vi "Results_filename_checker.vi"(4 "Filelength":i32=25, 5 "Warn if Already Exists":bool, 6 "Comment":string, 7 "Show Error handler":bool=TRUE, 8 "Results file":path) -> (0 "exists?":bool, 1 "Error String":string, 2 "cancelled":bool, 3 "Results file output":path)   [LabVIEW 2010]
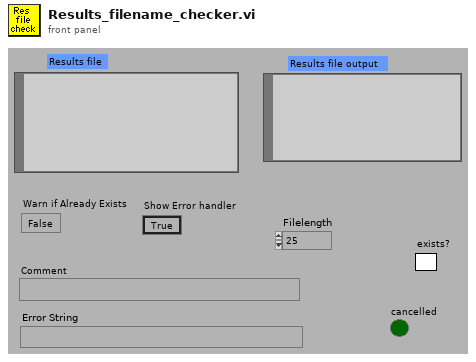
[diagram p1: front panel]
types:
  T1 = enum32{"existing file", "new file", "new or existing file", "existing dir", "new dir", "new or existing dir", "existing file (use LLBs)", "new file (use LLBs)", "new or existing file (use LLBs)", "new or existing file or directory (use LLBs)"}
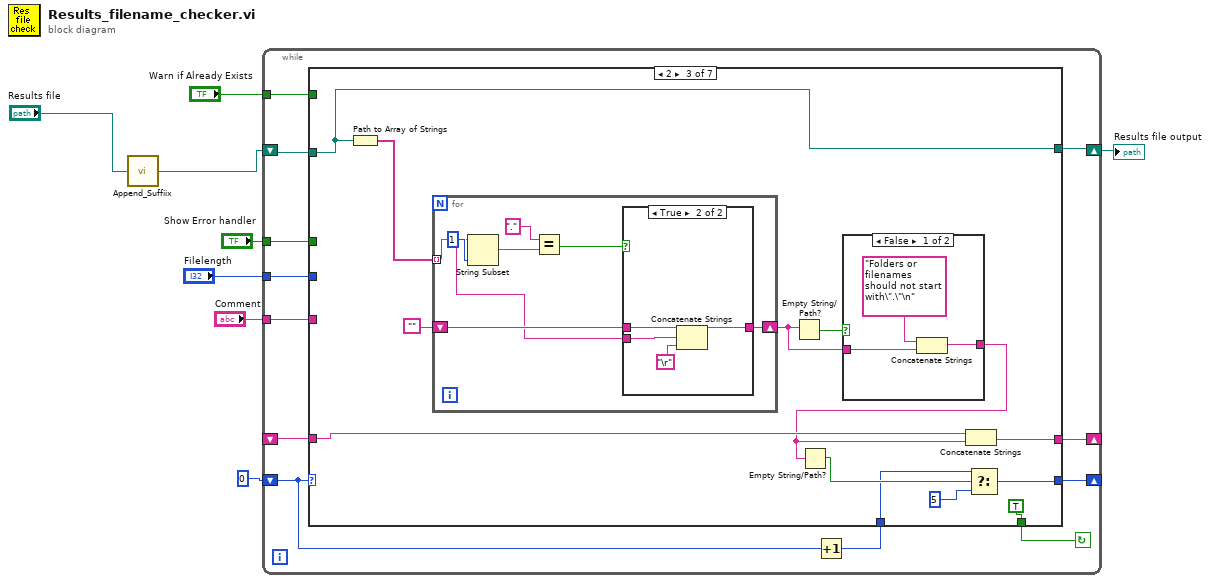
[diagram p0: block diagram]
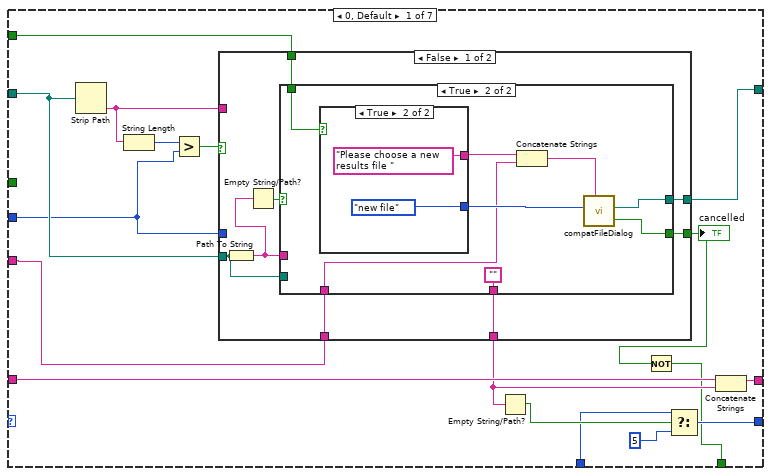
[diagram p2: hidden frame]
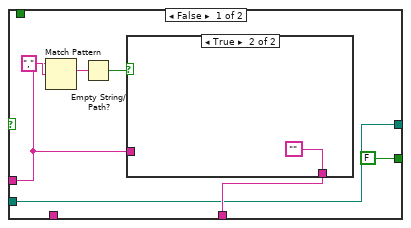
[diagram p3: hidden frame]
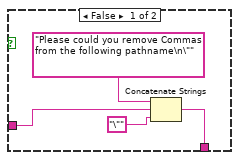
[diagram p4: hidden frame]
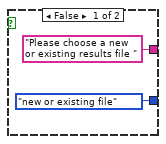
[diagram p5: hidden frame]
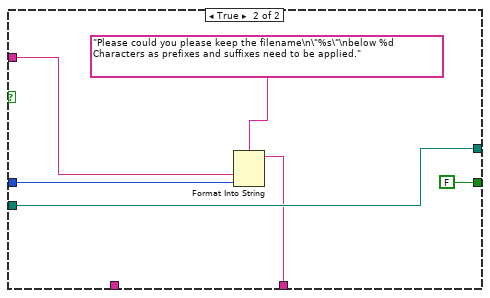
[diagram p6: hidden frame]
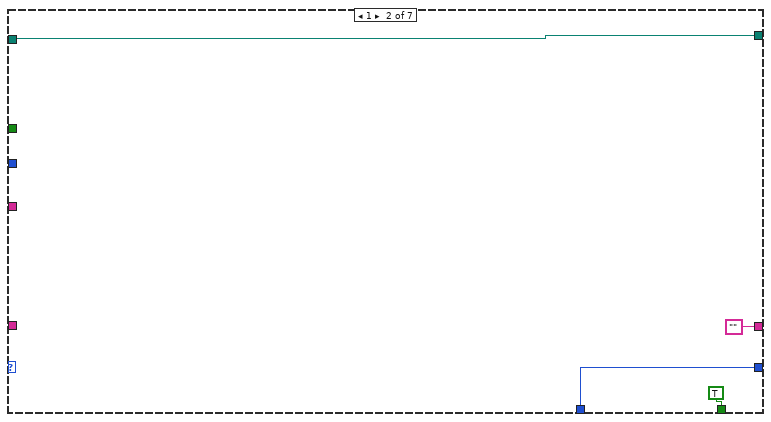
[diagram p7: hidden frame]
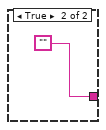
[diagram p8: hidden frame]
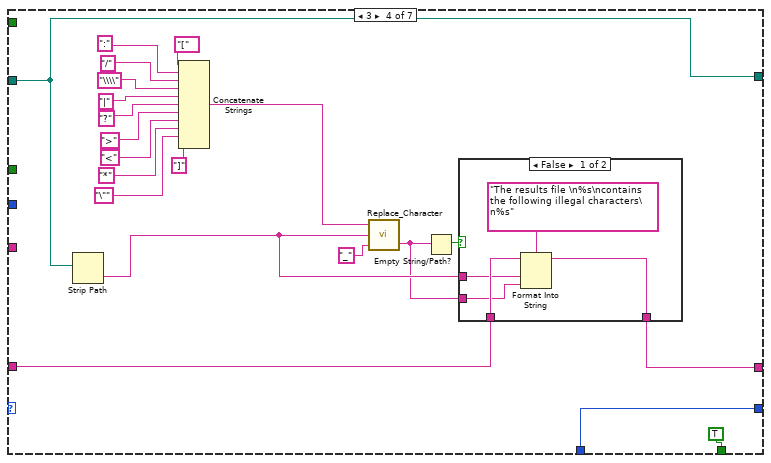
[diagram p10: hidden frame]
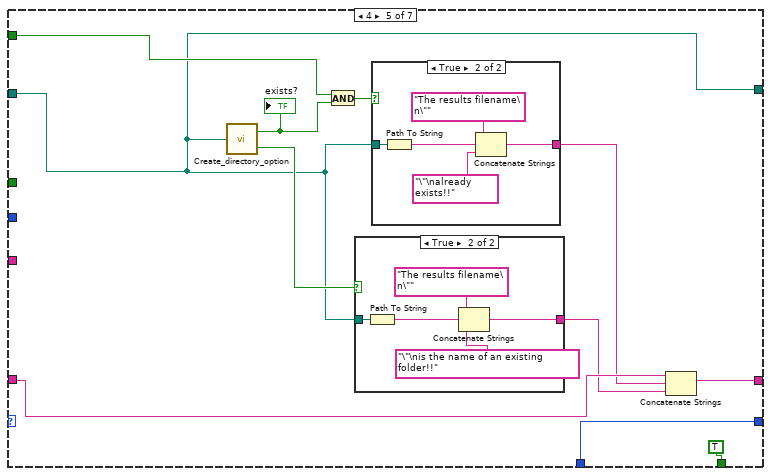
[diagram p12: hidden frame]
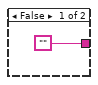
[diagram p13: hidden frame]
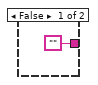
[diagram p14: hidden frame]
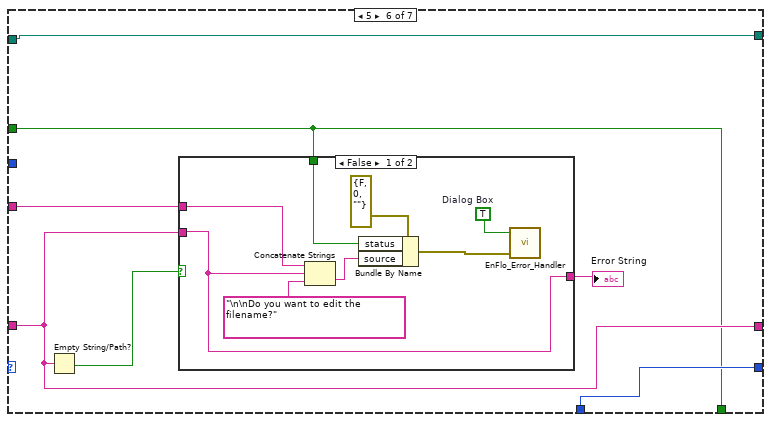
[diagram p15: hidden frame]
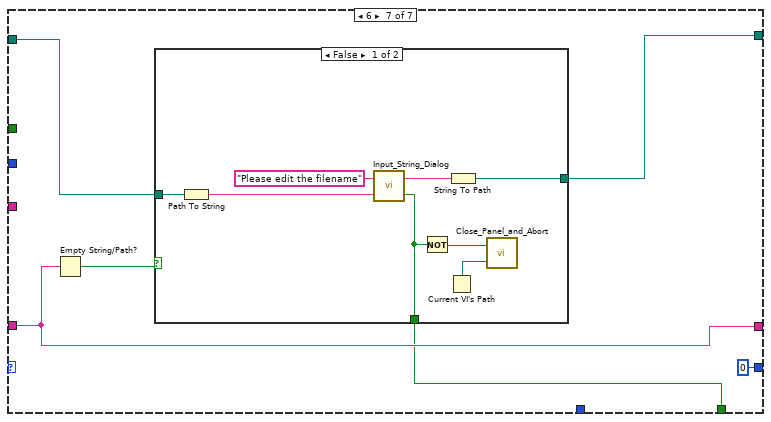
[diagram p17: hidden frame]
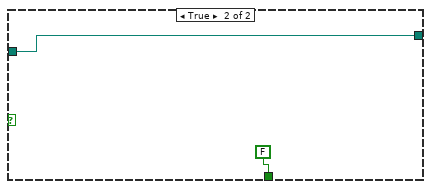
[diagram p18: hidden frame]
diagram:
  n1 = call "Append_Suffiix.vi"("Results file"="Results file") -> ("appended path"=w1:path)
  n2 = while {
    shift-left: 0 -> [w16]
    shift-right: [w12] -> _
    shift-left: _ -> [w15]
    shift-right: [w14] -> _
    tunnel: "Show Error handler" -> [w17]
    shift-left: w1 -> [w20]
    shift-right: [w19] -> w8
    tunnel: "Warn if Already Exists" -> [w11]
    tunnel: "Comment" -> [w10]
    tunnel: "Filelength" -> [w9]
    stop <- w18 continue-if-true
    n3 = Increment(x=w16) -> (x+1=w13:i32)
    n4 = case shown="2" w16 {
      tunnel: w20 -> [w26 w76 w80 w116 w136 w160 w179]
      tunnel: [w27 w76 w80 w116 w136 w160 w180] -> w19
      tunnel: [w23 TRUE ("Ok Out") TRUE ("Ok Out") TRUE ("Ok Out") TRUE ("Ok Out") w161 w177] -> w18
      tunnel: w17 -> [_ _ _ _ _ w161 _]
      tunnel: w15 -> [w36 _ w85 w114 w143 w163 w178]
      tunnel: [w35 "" w83 w113 w142 w163 w178] -> w14
      tunnel: w13 -> [w32 w78 w82 w112 w140 w162 _]
      tunnel: [w30 w78 w81 w112 w140 w162 0 ("f")] -> w12
      tunnel: w11 -> [w25 _ _ _ w137 _ _]
      tunnel: w10 -> [w22 _ _ _ _ w159 _]
      tunnel: w9 -> [w21 _ _ _ _ _ _]
      frame 0, Default {
        n5 = Strip Path(path=w26) -> (name=w29:string)  [unwired: 1 out]
        n6 = String Length(string=w29) -> (length=w28:i32)
        n7 = Greater?(x=w28, y=w21) -> (0:w37:bool)
        n8 = case shown="False" w37 {
          tunnel: w26 -> [w41 w75]
          tunnel: w29 -> [_ w73]
          tunnel: [w45 w71] -> w34
          tunnel: [w42 w75] -> w27
          tunnel: w25 -> [w40 _]
          tunnel: [w39 FALSE ("cancelled")] -> w24
          tunnel: w22 -> [w38 _]
          tunnel: w21 -> [_ w72]
          frame False {
            n9 = Path To String(path=w41) -> (string=w44:string)
            n10 = Empty String/Path?(string/path=w44) -> (empty?=w43:bool)
            n11 = case shown="True" w43 {
              tunnel: [w52 ""] -> w45
              tunnel: w44 -> [w48 _]
              tunnel: [w47 w65] -> w42
              tunnel: w41 -> [w47 _]
              tunnel: w40 -> [_ w63]
              tunnel: [FALSE ("cancelled") w61] -> w39
              tunnel: w38 -> [_ w59]
              frame False {
                n12 = Match Pattern(string=w48, regular expression=",") -> (match substring=w50:string)  [unwired: 4 out]
                n13 = Empty String/Path?(string/path=w50) -> (empty?=w49:bool)
                n14 = case shown="True" w49 {
                  tunnel: w48 -> [w55 _]
                  tunnel: [w54 ""] -> w52
                  frame False {
                    n15 = Concatenate Strings("Please could you remove Commas from the following pathname\n\"", w55, "\"") -> (w54:string)
                  }
                  frame True {
                  }
                }
              }
              frame True {
                n16 = case shown="True" w63 {
                  tunnel: [T1."new or existing file" ("f") T1."new file" ("select mode (2)")] -> w62
                  tunnel: ["Please choose a new or existing results file " ("prompt") "Please choose a new results file " ("prompt")] -> w60
                  frame False {
                  }
                  frame True {
                  }
                }
                n17 = Concatenate Strings(w60, w59) -> (w58:string)
                n18 = call <vilib>:"compatFileDialog.vi"("prompt"=w58, "select mode (2)"=w62) -> ("cancelled"=w61:bool, "path"=w65:path)  [unwired: 5 in, 3 out]
              }
            }
          }
          frame True {
            n19 = Format Into String(format string="Please could you please keep the filename\n\"%s\"\nbelow %d Characters as prefixes and suffixes need to be applied.", w73, w72) -> (resulting string=w71:string)  [unwired: 2 in, 1 out]
          }
        }
        "cancelled" <- w24
        n20 = Empty String/Path?(string/path=w34) -> (empty?=w33:bool)
        n21 = Not(x=w24) -> (.not. x?=w23:bool)
        n22 = Select(t=w32, s=w33, f=5) -> (s? t:f=w30:i32)
        n23 = Concatenate Strings(w36, w34) -> (w35:string)
      }
      frame 1 {
      }
      frame 2 {
        n24 = Path to Array of Strings(0:w80) -> (2:w90:string[])  [unwired: 1 out]
        n25 = for {
          tunnel: w90 -> [w98] mode=indexing
          shift-right: [w97] -> w88
          shift-left: "" -> [w99]
          n26 = String Subset(string=w98, length (rest)=1 ("length")) -> (substring=w102:string)  [unwired: 1 out]
          n27 = Equal?(x=".", y=w102) -> (x = y?=w100:bool)
          n28 = case shown="True" w100 {
            tunnel: w99 -> [w104 w108]
            tunnel: w98 -> [_ w107]
            tunnel: [w104 w106] -> w97
            frame False {
            }
            frame True {
              n29 = Concatenate Strings(w108, w107, "\r") -> (w106:string)
            }
          }
        }
        n30 = Empty String/Path?(string/path=w88) -> (empty?=w89:bool)
        n31 = case shown="False" w89 {
          tunnel: [w93 ""] -> w84
          tunnel: w88 -> [w94 _]
          frame False {
            n32 = Concatenate Strings("Folders or filenames should not start with\".\"\n", w94) -> (w93:string)
          }
          frame True {
          }
        }
        n33 = Empty String/Path?(string/path=w84) -> (empty?=w87:bool)
        n34 = Concatenate Strings(w85, w84) -> (w83:string)
        n35 = Select(t=w82, s=w87, f=5) -> (s? t:f=w81:i32)
      }
      frame 3 {
        n36 = Strip Path(path=w116) -> (name=w110:string)  [unwired: 1 out]
        n37 = Concatenate Strings("[" ("Substring"), ":", "/", "\\\\", "|", "?", ">", "<", "*", "\"", "]" ("Substring")) -> (w118:string)
        n38 = call "Replace_Character.vi"("Replace with"="_", "Input String"=w110, "Search For"=w118) -> ("Matched Characters"=w109:string)  [unwired: 1 out]
        n39 = Empty String/Path?(string/path=w109) -> (empty?=w115:bool)
        n40 = case shown="False" w115 {
          tunnel: w114 -> [w133 w135]
          tunnel: [w132 w135] -> w113
          tunnel: w110 -> [w131 _]
          tunnel: w109 -> [w130 _]
          frame False {
            n41 = Format Into String(format string="The results file \n%s\ncontains the following illegal characters\n%s" ("Format String"), initial string=w133, w131, w130) -> (resulting string=w132:string)  [unwired: 1 in, 1 out]
          }
          frame True {
          }
        }
      }
      frame 4 {
        n42 = call "Create_directory_option.vi"("Filename"=w136) -> ("Path is to existing File"=w145:bool, "Path is to existing Directory"=w138:bool)
        "exists?" <- w145
        n43 = And(x=w137, y=w145) -> (x .and. y?=w144:bool)
        n44 = case shown="True" w138 {
          tunnel: w136 -> [_ w150]
          tunnel: ["" w149] -> w139
          frame False {
          }
          frame True {
            n45 = Path To String(path=w150) -> (string=w148:string)
            n46 = Concatenate Strings("The results filename\n\"", w148, "\"\nis the name of an existing folder!!") -> (w149:string)
          }
        }
        n47 = case shown="True" w144 {
          tunnel: w136 -> [_ w156]
          tunnel: ["" w155] -> w141
          frame False {
          }
          frame True {
            n48 = Path To String(path=w156) -> (string=w154:string)
            n49 = Concatenate Strings("The results filename\n\"", w154, "\"\nalready exists!!") -> (w155:string)
          }
        }
        n50 = Concatenate Strings(w143, w141, w139) -> (w142:string)
      }
      frame 5 {
        n51 = Empty String/Path?(string/path=w163) -> (empty?=w165:bool)
        n52 = case shown="False" w165 {
          tunnel: w163 -> [w167 w174]
          tunnel: [w167 w174] -> w164
          tunnel: w161 -> [w169 _]
          tunnel: w159 -> [w166 _]
          frame False {
            w171 = TRUE  # Dialog Box
            n53 = Concatenate Strings(w166, w167, "\n\nDo you want to edit the filename?") -> (w168:string)
            n54 = Bundle By Name(cluster=errorcluster {"status"=FALSE, "code"=0, "source"=""} ("error in (no error)"), "status"=w169, "source"=w168) -> (w172:errorcluster)
            n55 = call "EnFlo_Error_Handler.vi"("error in (no error)"=w172, "Dialog Box (T)"=w171) -> ()  [unwired: 1 in, 3 out]
          }
          frame True {
          }
        }
        "Error String" <- w164
      }
      frame 6 {
        n56 = Empty String/Path?(string/path=w178) -> (empty?=w175:bool)
        n57 = case shown="False" w175 {
          tunnel: [w181 w189] -> w180
          tunnel: [w183 FALSE ("Ok Out")] -> w177
          tunnel: w179 -> [w186 w189]
          frame False {
            n58 = Path To String(path=w186) -> (string=w182:string)
            n59 = call "Input_String_Dialog.vi"("Value"=w182, "Message to user"="Please edit the filename") -> ("Ok Out"=w183:bool, "Output string"=w187:string)
            n60 = Not(x=w183) -> (.not. x?=w185:bool)
            n61 = Current VI's Path() -> (path=w184:path)
            n62 = String To Path(string=w187) -> (path=w181:path)
            n63 = call "Close_Panel_and_Abort.vi"("Vi path"=w184, "stop"=w185) -> ()  [unwired: 1 out]
          }
          frame True {
          }
        }
      }
    }
  }
  "Results file output" <- w8
